vi "CreateSlide.vi"(8 "error in (no error)":errorcluster, 9 "Type (FP)":T1=enum."FP", 10 "Path":path) -> (0 "error out":errorcluster, 3 "BD Slide":refnum<class "Slide.lvclass">)   [LabVIEW 2017, in "Slide.lvclass"]
uses:
  Slide.lvclass
  SlideType.ctl
  Slide.lvclass/Slide.ctl
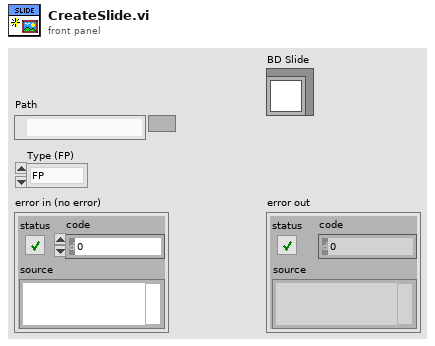
[diagram p1: front panel]
types:
  T1 = typedef "Slide.lvclass/SlideType.ctl" = enum16{"Image", "FP", "BD"}
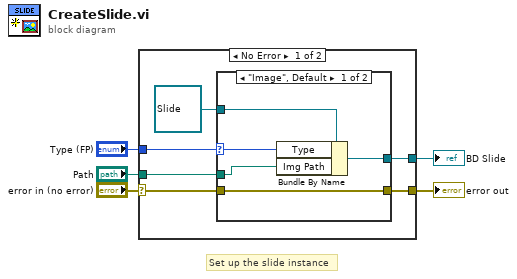
[diagram p0: block diagram]
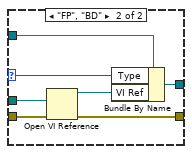
[diagram p2: hidden frame]
diagram:
  # "Set up the slide instance"
  n1 = case shown="No Error" "error in (no error)" {
    selector: "error in (no error)" -> [w7 w24]
    tunnel: [w6 w24] -> w4
    tunnel: [w10 _] -> w3
    tunnel: "Type (FP)" -> [w9 _]
    tunnel: "Path" -> [w8 _]
    frame No Error {
      n2 = case shown="\"Image\", Default" w9 {
        selector: w9 -> [w14 w20]
        tunnel: refnum<class "Slide.lvclass"> refnum ("Slide.lvclass") -> [w15 w22]
        tunnel: [w16 w21] -> w10
        tunnel: w8 -> [w13 w19]
        tunnel: w7 -> [w12 w18]
        tunnel: [w12 w17] -> w6
        frame "Image", Default {
          n3 = Bundle By Name(cluster=w15, "Type"=w14, "Img Path"=w13) -> (w16:refnum<class "Slide.lvclass">)
        }
        frame "FP", "BD" {
          n4 = Open VI Reference(vi path=w19, error in (no error)=w18) -> (vi reference=w23:refnum<vi>, error out=w17:errorcluster)  [unwired: 4 in]
          n5 = Bundle By Name(cluster=w22, "Type"=w20, "VI Ref"=w23) -> (w21:refnum<class "Slide.lvclass">)
        }
      }
    }
    frame Error {
    }
  }
  "BD Slide" <- w3
  "error out" <- w4
